vi "Initialize.vi"(7 "Parcel Weight [kg]":dbl, 8 "error in (no error)":errorcluster, 9 "Recipient Data":T1, 10 "Sender Data":T1, 11 "Post in":refnum<class "Post.lvclass">) -> (0 "error out":errorcluster, 3 "Post out":refnum<class "Post.lvclass">)   [LabVIEW 2019, in "Post.lvclass"]
uses:
  Post.lvclass
  C:/Users/Extensa/Desktop/Fabryka/Fabryka Rozwiazanie/Delivery/Delivery/Delivery.lvclass
  Controls/#cluster_PersonalData.ctl
  Delivery/Delivery.lvclass/Delivery.ctl
  Delivery/Delivery.lvclass
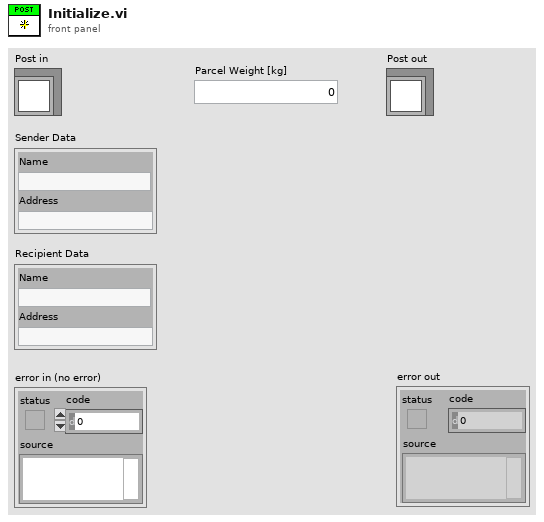
[diagram p1: front panel]
types:
  T1 = typedef "#cluster_PersonalData.ctl" = cluster{"Name":string, "Address":string}
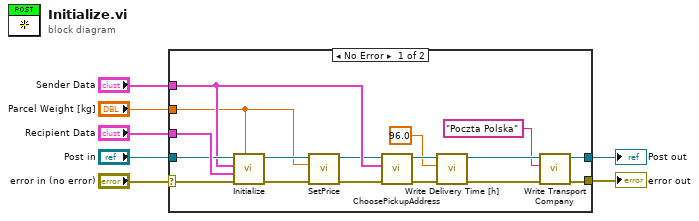
[diagram p0: block diagram]
diagram:
  n1 = case shown="No Error" "error in (no error)" {
    selector: "error in (no error)" -> [w24 w25]
    tunnel: "Recipient Data" -> [w23 _]
    tunnel: "Post in" -> [w22 w26]
    tunnel: "Sender Data" -> [w21 _]
    tunnel: [w11 w26] -> w3
    tunnel: [w10 w25] -> w2
    tunnel: "Parcel Weight [kg]" -> [w16 _]
    frame No Error {
      n2 = call-parent "Initialize.vi"("Parcel Weight [kg]"=w16, "error in (no error)"=w24, "Recipient Data"=w23, "Sender Data"=w21, "Delivery in"=w22) -> ("error out"=w20:errorcluster, "Delivery out"=w17:refnum<class "Post.lvclass">)  [unwired: 5 in]
      n3 = call "SetPrice.vi"("error in (no error)"=w20, "Parcel Weight [kg]"=w16, "Post in"=w17) -> ("error out"=w19:errorcluster, "Post out"=w18:refnum<class "Post.lvclass">)  [unwired: 7 in]
      n4 = call "ChoosePickupAddress.vi"("error in (no error)"=w19, "Sender Data"=w21, "Post in"=w18) -> ("error out"=w14:errorcluster, "Post out"=w15:refnum<class "Post.lvclass">)  [unwired: 7 in]
      n5 = call "Write Delivery Time [h].vi"("error in (no error)"=w14, "Delivery Time [h]"=96.0, "Delivery in"=w15) -> ("error out"=w13:errorcluster, "Delivery out"=w12:refnum<class "Post.lvclass">)  [unwired: 7 in]
      n6 = call "Write Transport Company.vi"("error in (no error)"=w13, "Transport Company"="Poczta Polska", "Delivery in"=w12) -> ("error out"=w10:errorcluster, "Delivery out"=w11:refnum<class "Post.lvclass">)  [unwired: 7 in]
    }
    frame Error {
    }
  }
  "error out" <- w2
  "Post out" <- w3
